vi "SV Aures Sharpness_2014.vi"   [LabVIEW 2017, in "SoundVib_SoundQuality.lvlib"]
doc: "Computes sharpness from the sound pressure signal waveform, the 1/3-octave band spectrum calculated over the frequency range 25 Hz to 12.5 kHz, or the specific loudness that the SV Stationary Loudness VI returns. Wire data to the <B>sound pressure signal [Pa]</B> input to determine the polymorphic instance to use or manually select the instance."
uses:
  <vilib>/addons/Sound and Vibration/svt_Sound Quality/SoundVib_SoundQuality.lvlib
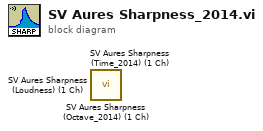
[diagram p0: block diagram]
diagram:
  n1 = call <vilib>:"SV Aures Sharpness (Octave_2014) (1 Ch).vi"() -> ()  [unwired: 12 in, 4 out]
  n2 = call <vilib>:"SV Aures Sharpness (Time_2014) (1 Ch).vi"() -> ()  [unwired: 12 in, 4 out]
  n3 = call <vilib>:"SV Aures Sharpness (Loudness) (1 Ch).vi"() -> ()  [unwired: 12 in, 4 out]
